vi "Periodic Tasks.vi"(8 "error in":errorcluster) -> ()   [LabVIEW 2017]
doc: "This VI runs in parallel to other tasks. It can contain as many user-defined periodic loops as you need. These can carry out PID or other sorts of timed response."
uses:
  <vilib>/Rock Robotics/WPI/Utilities/WPI_GetSetVariantRefNum.vi
  Robot Global Data.vi
  <vilib>/Rock Robotics/Network Tables/NT Write Number.vi
  <vilib>/Rock Robotics/SystemInterfaces/AI/FPGA_AIChannel.ctl
  <vilib>/Rock Robotics/WPI/Ultrasonic/WPI_SonarMB1010AnalogGetRange.vi
  <vilib>/Rock Robotics/WPI/Ultrasonic/WPI_SonarMB1010AnalogClose.vi
  <vilib>/Rock Robotics/WPI/Ultrasonic/WPI_SonarMB1010AnalogOpen.vi
  <vilib>/Rock Robotics/WPI/Ultrasonic/WPI_SonarMB1010AnalogRefNum Registry Set.vi
panel:
  out "Time Delta(ms)":u32
  in  "Reset Time":bool
  out "Elapsed Time":u32
  out "Time(sec)":dbl
  out "nAVX":T1
  out "distance":dbl(slide)=125.0 scale=0.0..250.0 scale format="%3d"
  in  "Scaling Factor":dbl=0.025
  in  "Average Bits":u8=3 max=15
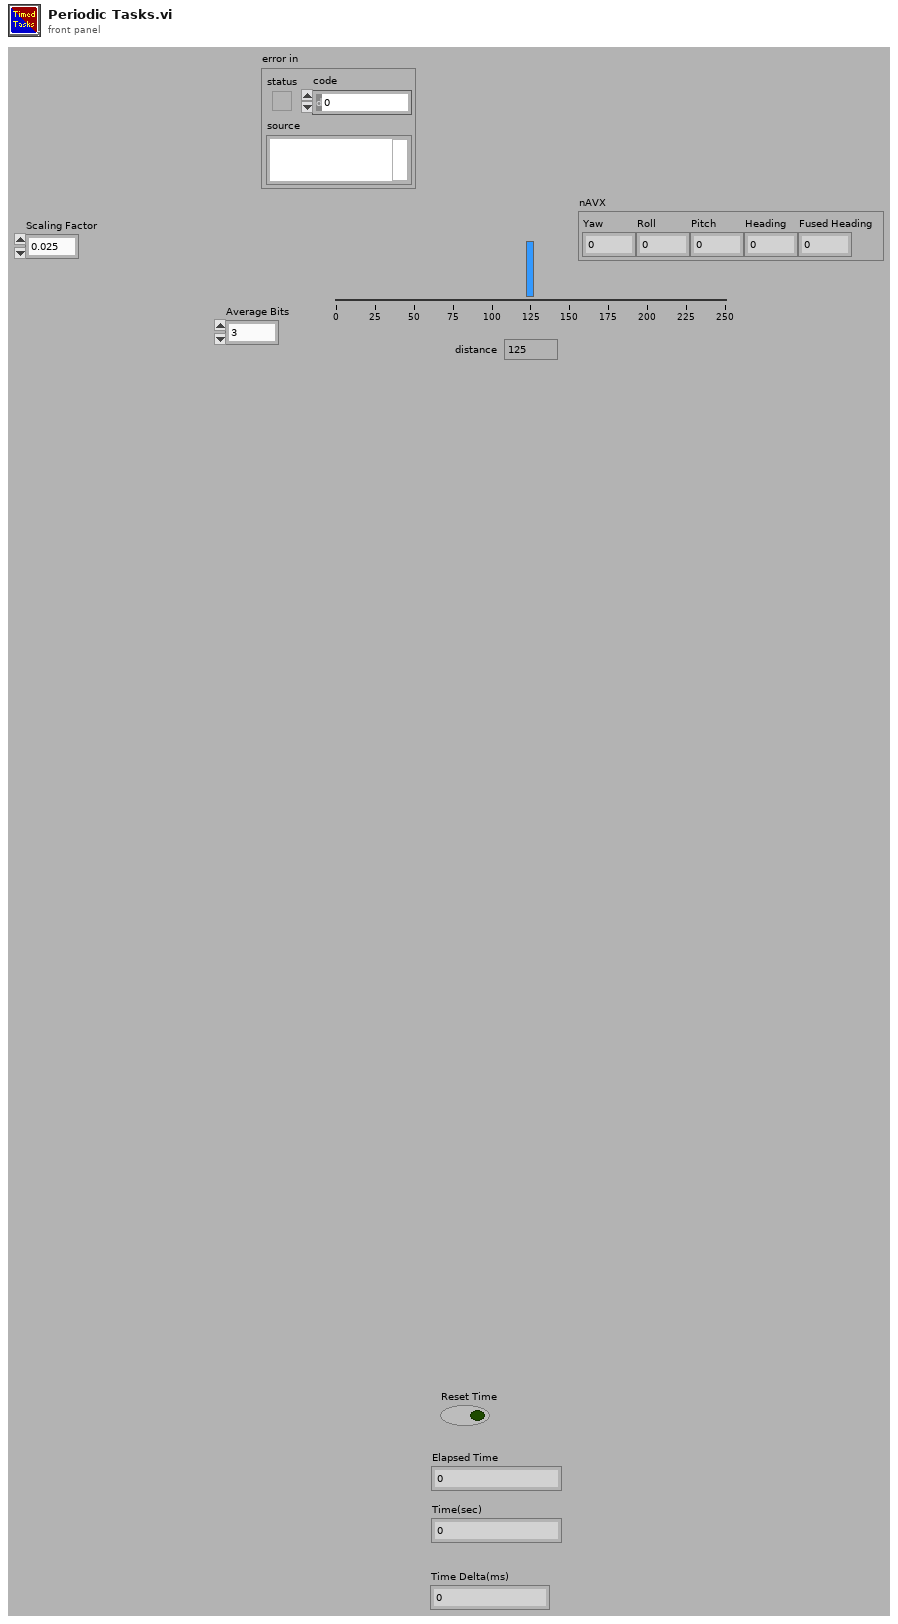
[diagram p1: front panel]
types:
  T1 = cluster{"Yaw":dbl, "Roll":dbl, "Pitch":dbl, "Heading":dbl, "Fused Heading":dbl}
  T2 = typedef "WPI_JoystickDevRef.ctl" = cluster{"Device":T3}
  T3 = typedef "WPI_JoystickDeviceEnum.ctl" = enum16{"USB 0", "USB 1", "USB 2", "USB 3", "USB 4", "USB 5"}
  T4 = typedef "WPI_RobotDriveDevRef.ctl" = cluster{"DevStatus":errorcluster, "Motors[]":T5[], "Square Inputs":bool, "Max Output":dbl}
  T5 = typedef "WPI_MotorControlDeviceRef.ctl" = cluster{"DeviceStatus":errorcluster, "Type":T6, "PWM":cluster{"PWM Channel":T7, "DeadBand":T8}, "CAN":cluster{"Device Number":u8, "SetOutput VI Ref":variant, "GetOutput VI Ref":variant, "Enable VI Ref":variant, "Disable VI Ref":variant, "Data":variant}, "Invert":bool, "DIO PWM":cluster{"PWM \"Enable\" Channel":T7, "DIOChannel":T9, "PWM Rate":dbl}}
  T6 = typedef "WPI_MotorControlType.ctl" = enum16{"PWM", "CAN", "DIO PWM"}
  T7 = typedef "FPGA_DIOPWMChannel.ctl" = enum8{"PWM 0", "PWM 1", "PWM 2", "PWM 3", "PWM 4", "PWM 5", "PWM 6", "PWM 7", "PWM 8", "PWM 9", "PWM MXP 0", "PWM MXP 1", "PWM MXP 2", "PWM MXP 3", "PWM MXP 4", "PWM MXP 5", "PWM MXP 6", "PWM MXP 7", "PWM MXP 8", "PWM MXP 9", "Invalid"}
  T8 = typedef "WPI_PWMDeadband.ctl" = cluster{"Name":string, "maxPositivePwm":i32, "minPositivePwm":i32, "centerPwm":i32, "maxNegativePwm":i32, "minNegativePwm":i32, "angularRange":u16}
  T9 = typedef "FPGA_DIOChannel.ctl" = enum8{"DIO 0", "DIO 1", "DIO 2", "DIO 3", "DIO 4", "DIO 5", "DIO 6", "DIO 7", "DIO 8", "DIO 9", "DIO MXP 0", "DIO MXP 1", "DIO MXP 2", "DIO MXP 3", "DIO MXP 4", "DIO MXP 5", "DIO MXP 6", "DIO MXP 7", "DIO MXP 8", "DIO MXP 9", "DIO MXP 10", "DIO MXP 11", "DIO MXP 12", "DIO MXP 13", "DIO MXP 14", "DIO MXP 15", "SPI Port CS1", "SPI Port CS2", "SPI Port CS3", "SPI Port MISO", "SPI Port MOSI", "Invalid"}
  T10 = typedef "FPGA_AIChannel.ctl" = enum8{"AI 0", "AI 1", "AI 2", "AI 3", "AI MXP 0", "AI MXP 1", "AI MXP 2", "AI MXP 3", "Invalid"}
  T11 = typedef "WPI_SonarMB1010AnalogDeviceRef.ctl" = cluster{"AIDeviceRef":T12, "Scaling factor (V/in)":dbl, "Average Bits":u8}
  T12 = typedef "WPI_AnalogChannelDevRef.ctl" = cluster{"DevStatus":errorcluster, "Analog Channel":T10}
  T13 = cluster{"JoystickDevRef":T2, "RobotDriveDevRef":T4}
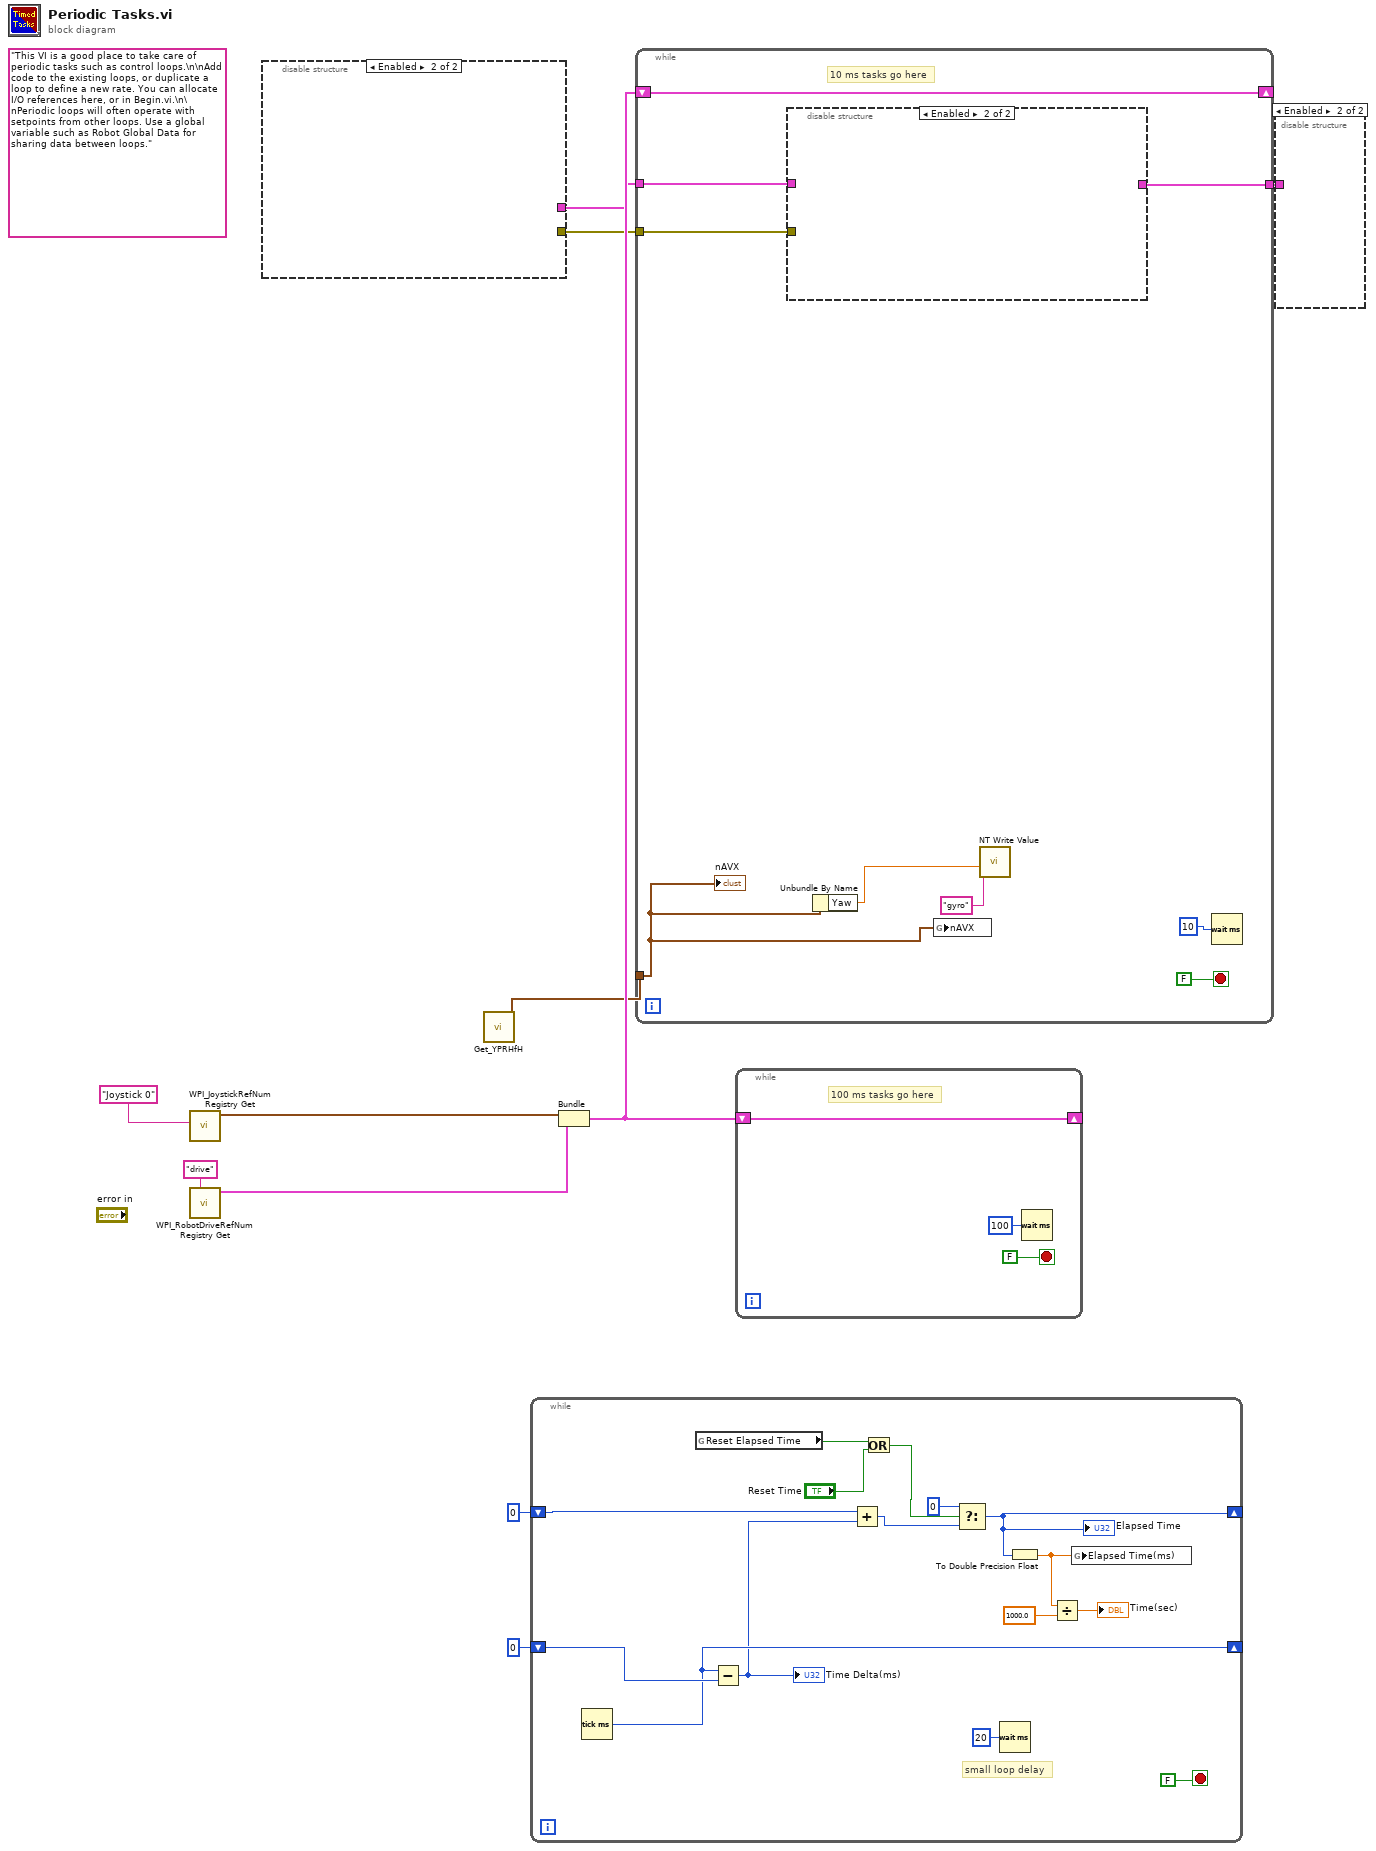
[diagram p0: block diagram]
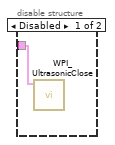
[diagram p2: hidden frame]
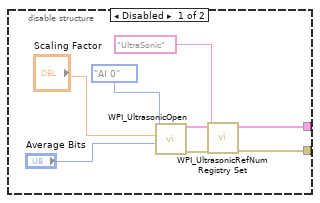
[diagram p3: hidden frame]
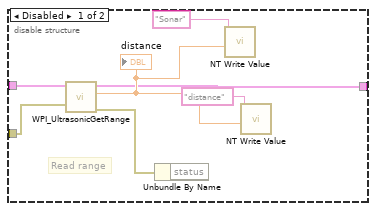
[diagram p4: hidden frame]
diagram:
  (unwired) "This VI is a good place to take care of periodic tasks such as control loops.\n\nAdd code to the existing loops, or duplicate a loop to define a new rate. You can allocate I/O references here, or in Begin.vi.\n\nPeriodic loops will often operate with setpoints from other loops. Use a global variable such as Robot Global Data for sharing data between loops."
  n1 = call <vilib>:"WPI_JoystickRefNum Registry Get.vi"("refnum name"="Joystick 0") -> ("JoystickDevRef"=w9:T2)  [unwired: 1 in, 9 out]
  n2 = call <vilib>:"WPI_RobotDriveRefNum Registry Get.vi"("refnum name"="drive") -> ("RobotDriveDevRef"=w8:T4)  [unwired: 1 in, 9 out]
  n3 = disable-structure shown="Enabled" {
    disable-tunnel: [w13 _] -> w6
    disable-tunnel: [w12 _] -> w5
    frame Disabled {
      n4 = call-poly <vilib>:"WPI_UltrasonicOpen.vi"("Average Bits"="Average Bits", "Scaling factor (V/in)"="Scaling Factor", "Analog Channel"=FPGA_AIChannel."AI 0") -> ("error out"=w17:errorcluster, "SonarMB1010AnalogDevRef"=w15:T11)  [unwired: 7 in]
      n5 = call-poly <vilib>:"WPI_UltrasonicRefNum Registry Set.vi"("error in (no error)"=w17, "refnum name"="UltraSonic", "SonarMB1010AnalogDevRef"=w15) -> ("error out"=w12:errorcluster, "SonarMB1010AnalogDevRef"=w13:T11)  [unwired: 7 in]
    }
    frame Enabled {
    }
  }
  n6 = call <vilib>:"Get_YPRHfH.vi"() -> ("YRPHfH"=w3:T1)  [unwired: 11 in]
  n7 = while {
    shift-right: [w21] -> _
    shift-left: u32 0 ("millisecond timer value") -> [w32]
    shift-right: [w28] -> _
    shift-left: u32 0 -> [w30]
    stop <- FALSE stop-if-true
    # "small loop delay"
    n8 = Tick Count (ms)() -> (millisecond timer value=w21:u32)
    n9 = global read "Robot Global Data.vi" "Reset Elapsed Time"() -> (w27:bool)
    n10 = Subtract(x=w21, y=w32) -> (x-y=w20:u32)
    "Time Delta(ms)" <- w20
    n11 = Add(x=w30, y=w20) -> (x+y=w31:u32)
    n12 = Or(x=w27, y="Reset Time") -> (x .or. y?=w22:bool)
    n13 = Select(t=u32 0, s=w22, f=w31) -> (s? t:f=w28:u32)
    "Elapsed Time" <- w28
    n14 = Wait (ms)(milliseconds to wait=u32 20) -> ()  [unwired: 1 out]
    n15 = To Double Precision Float(number=w28) -> (double precision float=w25:dbl)
    n16 = Divide(x=w25, y=1000.0) -> (x/y=→"Time(sec)":dbl)
    n17 = global write "Robot Global Data.vi" "Elapsed Time(ms)"(w25) -> ()
  }
  n18 = Bundle("JoystickDevRef"=w9, "RobotDriveDevRef"=w8) -> (w7:T13)  [unwired: 1 out]
  n19 = while {
    shift-right: [w41] -> _
    shift-left: w7 -> [w41]
    tunnel: w6 -> [w40]
    tunnel: w5 -> [w39]
    tunnel: [w38] -> w4
    tunnel: w3 -> [w37]
    stop <- FALSE stop-if-true
    # "10 ms tasks go here"
    n20 = disable-structure shown="Enabled" {
      disable-tunnel: w40 -> [w46 _]
      disable-tunnel: w39 -> [w45 _]
      disable-tunnel: [w44 _] -> w38
      frame Disabled {
        # "Read range"
        n21 = call-poly <vilib>:"WPI_UltrasonicGetRange.vi"("error in"=w45, "SonarMB1010AnalogDevRef"=w46) -> ("error out"=w50:errorcluster, "Distance"=w48:dbl, "SonarMB1010AnalogDevRef"=w44:T11)  [unwired: 7 in]
        "distance" <- w48
        n22 = Unbundle By Name(w50) -> ()  [unwired: 1 out]
        n23 = call-poly <vilib>:"NT Write Value.vi"("Numeric"=w48, "Name"="Sonar") -> ()  [unwired: 9 in, 1 out]
        n24 = call-poly <vilib>:"NT Write Value.vi"("Numeric"=w48, "Name"="distance") -> ()  [unwired: 9 in, 1 out]
      }
      frame Enabled {
      }
    }
    n25 = Unbundle By Name(w37) -> ("Yaw"=w36:dbl)
    n26 = global write "Robot Global Data.vi" "nAVX"(w37) -> ()
    n27 = call-poly <vilib>:"NT Write Value.vi"("Numeric"=w36, "Name"="gyro") -> ()  [unwired: 9 in, 1 out]
    n28 = Wait (ms)(milliseconds to wait=u32 10) -> ()  [unwired: 1 out]
    "nAVX" <- w37
  }
  n29 = while {
    shift-right: [w51] -> _
    shift-left: w7 -> [w51]
    stop <- FALSE stop-if-true
    # "100 ms tasks go here"
    n30 = Wait (ms)(milliseconds to wait=u32 100) -> ()  [unwired: 1 out]
  }
  n31 = disable-structure shown="Enabled" {
    disable-tunnel: w4 -> [w54 _]
    frame Disabled {
      n32 = call-poly <vilib>:"WPI_UltrasonicClose.vi"("SonarMB1010AnalogDevRef"=w54) -> ()  [unwired: 10 in, 1 out]
    }
    frame Enabled {
    }
  }
